vi "HFRR ADV v013 new software.vi"() -> ()   [LabVIEW 2025] (continued)
              tunnel: [w2197] -> w2113 mode=indexing
              tunnel: [w2196] -> w2106 mode=indexing
              tunnel: w2150 -> [_]
              tunnel: [w2185] -> w2111 mode=indexing
              tunnel: [w2190] -> w2108 mode=indexing
              tunnel: [w2186] -> w2098 mode=indexing
              tunnel: [w2181] -> w2073 mode=indexing
              tunnel: [w2177] -> w2054 mode=indexing
              tunnel: [w2172] -> w2014 mode=indexing
              (unwired) 1.0 ("x")
              (unwired) TRUE ("line mode (F)")
              n2047 = Read from Text File "Read File"(file (use dialog)=w2208, error in=w2207) -> (text=w2173:string)  [unwired: 2 in, 3 out]
              n2048 = local write "String 12"(w2173) -> ()
              n2049 = String Subset(string=w2173, offset (0)=85, length (rest)=9 ("length (rest)")) -> (substring=w2175:string)
              n2050 = String Subset(string=w2173, offset (0)=35, length (rest)=9 ("length (rest)")) -> (substring=w2198:string)
              n2051 = String Subset(string=w2173, offset (0)=55, length (rest)=9 ("length (rest)")) -> (substring=w2183:string)
              n2052 = String Subset(string=w2173, offset (0)=25, length (rest)=9 ("length (rest)")) -> (substring=w2179:string)
              n2053 = String Subset(string=w2173, offset (0)=45, length (rest)=9 ("length (rest)")) -> (substring=w2188:string)
              n2054 = String Subset(string=w2173, offset (0)=15, length (rest)=9 ("length (rest)")) -> (substring=w2204:string)
              n2055 = String Subset(string=w2173, offset (0)=0, length (rest)=14 ("length (rest)")) -> (substring=w2201:string)
              n2056 = String Subset(string=w2173, offset (0)=65, length (rest)=9 ("length (rest)")) -> (substring=w2191:string)
              n2057 = Fract/Exp String To Number(string=w2175) -> (number=w2172:dbl)  [unwired: 3 in, 1 out]
              n2058 = Fract/Exp String To Number(string=w2198) -> (number=w2196:dbl)  [unwired: 3 in, 1 out]
              n2059 = Fract/Exp String To Number(string=w2183) -> (number=w2181:dbl)  [unwired: 3 in, 1 out]
              n2060 = Fract/Exp String To Number(string=w2179) -> (number=w2177:dbl)  [unwired: 3 in, 1 out]
              n2061 = Fract/Exp String To Number(string=w2188) -> (number=w2186:dbl)  [unwired: 3 in, 1 out]
              n2062 = Fract/Exp String To Number(string=w2204) -> (number=w2185:dbl)  [unwired: 3 in, 1 out]
              n2063 = Fract/Exp String To Number(string=w2201) -> (number=w2197:dbl)  [unwired: 3 in, 1 out]
              n2064 = Fract/Exp String To Number(string=w2191) -> (number=w2194:dbl)  [unwired: 3 in, 1 out]
              n2065 = Add(x=w2194, y=0.0) -> (x+y=w2190:dbl)
            }
            n2066 = Delete From Array(array=w2056, index=0) -> (array with subset deleted=w2029:dbl[])  [unwired: 1 in, 1 out]
            n2067 = Delete From Array(array=w2119, index=0) -> (array with subset deleted=w2092:dbl[])  [unwired: 1 in, 1 out]
            n2068 = Delete From Array(array=w2099, index=0) -> (array with subset deleted=w2087:dbl[])  [unwired: 1 in, 1 out]
            n2069 = Delete From Array(array=w2117, index=0) -> (array with subset deleted=w2118:dbl[])  [unwired: 1 in, 1 out]
            n2070 = call-poly <vilib>:"Mean.vi"("X"=w2029) -> ("mean"=→"КОФ2 4":dbl)  [unwired: 1 out]
            n2071 = call-poly <vilib>:"Mean.vi"("X"=w2092) -> ("mean"=→"КОФ3":dbl)  [unwired: 1 out]
            n2072 = call-poly <vilib>:"Mean.vi"("X"=w2087) -> ("mean"=→"CP3":dbl)  [unwired: 1 out]
            n2073 = Delete From Array(array=w2081, index=0) -> (array with subset deleted=w2008:dbl[])  [unwired: 1 in, 1 out]
            n2074 = Delete From Array(array=w2020, index=0) -> (array with subset deleted=w2007:dbl[])  [unwired: 1 in, 1 out]
            n2075 = Delete From Array(array=w2060, index=0) -> (array with subset deleted=w2031:dbl[])  [unwired: 1 in, 1 out]
            n2076 = Delete From Array(array=w2138, index=0) -> (array with subset deleted=w2093:dbl[])  [unwired: 1 in, 1 out]
            n2077 = Delete From Array(array=w2104, index=0) -> (array with subset deleted=w2089:dbl[])  [unwired: 1 in, 1 out]
            "array w/ subset deleted" <- w2089
            n2078 = Delete From Array(array=w2135, index=0) -> (array with subset deleted=w2136:dbl[])  [unwired: 1 in, 1 out]
            n2079 = call-poly <vilib>:"Mean.vi"("X"=w2031) -> ("mean"=→"КОФ2 2":dbl)  [unwired: 1 out]
            n2080 = call-poly <vilib>:"Mean.vi"("X"=w2093) -> ("mean"=→"КОФ1":dbl)  [unwired: 1 out]
            n2081 = Bundle "Bundle"(w2008, w2007) -> (w2013:cluster{dbl[], dbl[]})  [unwired: 1 in]
            n2082 = Bundle "Bundle"(w2008, w2136) -> (w2000:cluster{dbl[], dbl[]})  [unwired: 1 in]
            n2083 = Delete From Array(array=w2015, index=0) -> (array with subset deleted=w2003:dbl[])  [unwired: 1 in, 1 out]
            n2084 = Delete From Array(array=w2016, index=0) -> (array with subset deleted=w2005:dbl[])  [unwired: 1 in, 1 out]
            n2085 = Delete From Array(array=w2126, index=0) -> (array with subset deleted=w2127:dbl[])  [unwired: 1 in, 1 out]
            n2086 = Delete From Array(array=w2014, index=0) -> (array with subset deleted=w2001:dbl[])  [unwired: 1 in, 1 out]
            n2087 = Delete From Array(array=w2108, index=0) -> (array with subset deleted=w2109:dbl[])  [unwired: 1 in, 1 out]
            n2088 = Delete From Array(array=w2133, index=0) -> (array with subset deleted=w2039:dbl[])  [unwired: 1 in, 1 out]
            n2089 = Delete From Array(array=w2079, index=0) -> (array with subset deleted=w2035:dbl[])  [unwired: 1 in, 1 out]
            n2090 = Delete From Array(array=w2115, index=0) -> (array with subset deleted=w2037:dbl[])  [unwired: 1 in, 1 out]
            n2091 = Delete From Array(array=w2075, index=0) -> (array with subset deleted=w2033:dbl[])  [unwired: 1 in, 1 out]
            n2092 = Delete From Array(array=w2124, index=0) -> (array with subset deleted=w2038:dbl[])  [unwired: 1 in, 1 out]
            n2093 = Delete From Array(array=w2077, index=0) -> (array with subset deleted=w2034:dbl[])  [unwired: 1 in, 1 out]
            n2094 = Delete From Array(array=w2058, index=0) -> (array with subset deleted=w2030:dbl[])  [unwired: 1 in, 1 out]
            n2095 = Delete From Array(array=w2102, index=0) -> (array with subset deleted=w2088:dbl[])  [unwired: 1 in, 1 out]
            n2096 = Delete From Array(array=w2129, index=0) -> (array with subset deleted=w2090:dbl[])  [unwired: 1 in, 1 out]
            n2097 = Delete From Array(array=w2106, index=0) -> (array with subset deleted=w2036:dbl[])  [unwired: 1 in, 1 out]
            n2098 = Delete From Array(array=w2073, index=0) -> (array with subset deleted=w2032:dbl[])  [unwired: 1 in, 1 out]
            n2099 = Delete From Array(array=w2054, index=0) -> (array with subset deleted=w2028:dbl[])  [unwired: 1 in, 1 out]
            n2100 = Delete From Array(array=w2098, index=0) -> (array with subset deleted=w2086:dbl[])  [unwired: 1 in, 1 out]
            n2101 = Delete From Array(array=w2111, index=0) -> (array with subset deleted=w2091:dbl[])  [unwired: 1 in, 1 out]
            n2102 = Delete From Array(array=w2121, index=0) -> (array with subset deleted=w2004:dbl[])  [unwired: 1 in, 1 out]
            n2103 = Delete From Array(array=w2131, index=0) -> (array with subset deleted=w2006:dbl[])  [unwired: 1 in, 1 out]
            n2104 = Delete From Array(array=w2113, index=0) -> (array with subset deleted=w2002:dbl[])  [unwired: 1 in, 1 out]
            n2105 = Bundle "Bundle"(w2008, w2039) -> (w2026:cluster{dbl[], dbl[]})  [unwired: 1 in]
            n2106 = Bundle "Bundle"(w2008, w2093) -> (w2027:cluster{dbl[], dbl[]})  [unwired: 1 in]
            n2107 = Bundle "Bundle"(w2039, w2035) -> (w2041:cluster{dbl[], dbl[]})  [unwired: 1 in]
            n2108 = Bundle "Bundle"(w2004, w2003) -> (w2011:cluster{dbl[], dbl[]})  [unwired: 1 in]
            n2109 = Bundle "Bundle"(w2037, w2033) -> (w2043:cluster{dbl[], dbl[]})  [unwired: 1 in]
            n2110 = Bundle "Bundle"(w2004, w2037) -> (w2147:cluster{dbl[], dbl[]})  [unwired: 1 in]
            n2111 = Bundle "Bundle"(w2004, w2033) -> (w2071:cluster{dbl[], dbl[]})  [unwired: 1 in]
            n2112 = Bundle "Bundle"(w2004, w2092) -> (w2157:cluster{dbl[], dbl[]})  [unwired: 1 in]
            n2113 = Bundle "Bundle"(w2004, w2087) -> (w2095:cluster{dbl[], dbl[]})  [unwired: 1 in]
            n2114 = Bundle "Bundle"(w2004, w2118) -> (w2142:cluster{dbl[], dbl[]})  [unwired: 1 in]
            n2115 = Bundle "Bundle"(w2038, w2034) -> (w2042:cluster{dbl[], dbl[]})  [unwired: 1 in]
            n2116 = Bundle "Bundle"(w2006, w2005) -> (w2012:cluster{dbl[], dbl[]})  [unwired: 1 in]
            n2117 = Bundle "Bundle"(w2006, w2038) -> (w2149:cluster{dbl[], dbl[]})  [unwired: 1 in]
            n2118 = Bundle "Bundle"(w2006, w2034) -> (w2072:cluster{dbl[], dbl[]})  [unwired: 1 in]
            n2119 = Bundle "Bundle"(w2006, w2088) -> (w2096:cluster{dbl[], dbl[]})  [unwired: 1 in]
            n2120 = Bundle "Bundle"(w2006, w2090) -> (w2158:cluster{dbl[], dbl[]})  [unwired: 1 in]
            n2121 = Bundle "Bundle"(w2006, w2127) -> (w2140:cluster{dbl[], dbl[]})  [unwired: 1 in]
            n2122 = Bundle "Bundle"(w2036, w2032) -> (w2044:cluster{dbl[], dbl[]})  [unwired: 1 in]
            n2123 = Bundle "Bundle"(w2002, w2001) -> (w2010:cluster{dbl[], dbl[]})  [unwired: 1 in]
            n2124 = Bundle "Bundle"(w2002, w2036) -> (w2148:cluster{dbl[], dbl[]})  [unwired: 1 in]
            n2125 = Bundle "Bundle"(w2002, w2032) -> (w2070:cluster{dbl[], dbl[]})  [unwired: 1 in]
            n2126 = Bundle "Bundle"(w2002, w2086) -> (w2094:cluster{dbl[], dbl[]})  [unwired: 1 in]
            n2127 = Bundle "Bundle"(w2002, w2091) -> (w2156:cluster{dbl[], dbl[]})  [unwired: 1 in]
            n2128 = Bundle "Bundle"(w2002, w2109) -> (w2141:cluster{dbl[], dbl[]})  [unwired: 1 in]
            n2129 = call-poly <vilib>:"Mean.vi"("X"=w2089) -> ("mean"=→"CP1":dbl)  [unwired: 1 out]
            n2130 = call-poly <vilib>:"Mean.vi"("X"=w2030) -> ("mean"=→"КОФ2 3":dbl)  [unwired: 1 out]
            n2131 = call-poly <vilib>:"Mean.vi"("X"=w2088) -> ("mean"=→"CP2":dbl)  [unwired: 1 out]
            n2132 = call-poly <vilib>:"Mean.vi"("X"=w2090) -> ("mean"=→"КОФ2":dbl)  [unwired: 1 out]
            n2133 = call-poly <vilib>:"Mean.vi"("X"=w2028) -> ("mean"=→"КОФ2 5":dbl)  [unwired: 1 out]
            n2134 = call-poly <vilib>:"Mean.vi"("X"=w2086) -> ("mean"=→"CP4":dbl)  [unwired: 1 out]
            n2135 = call-poly <vilib>:"Mean.vi"("X"=w2091) -> ("mean"=→"КОФ4":dbl)  [unwired: 1 out]
            n2136 = Bundle "Bundle"(w2008, w2035) -> (w1999:cluster{dbl[], dbl[]})  [unwired: 1 in]
            n2137 = Bundle "Bundle"(w2008, w2089) -> (w2022:cluster{dbl[], dbl[]})  [unwired: 1 in]
            n2138 = Build Array "Build Array"(w1999, w2022) -> (w2025:cluster{dbl[], dbl[]}[])
            "XY Graph 17" <- w2025
            n2139 = Build Array "Build Array"(w2013, w2012, w2011, w2010) -> (→"Frequency ( Hz )":cluster{dbl[], dbl[]}[])
            n2140 = Build Array "Build Array"(w2041, w2042, w2043, w2044) -> (→"Air Temp ( °C ) vs Humidity ( % RH )":cluster{dbl[], dbl[]}[])
            n2141 = Build Array "Build Array"(w2026, w2149, w2147, w2148) -> (→"Air Temperature  ( °C )":cluster{dbl[], dbl[]}[])
            n2142 = Build Array "Build Array"(w1999, w2072, w2071, w2070) -> (→"Humidity ( %RH )":cluster{dbl[], dbl[]}[])
            n2143 = Build Array "Build Array"(w2027, w2158, w2157, w2156) -> (→"Coefficient Of Friction":cluster{dbl[], dbl[]}[])
            n2144 = Build Array "Build Array"(w2022, w2096, w2095, w2094) -> (→"Sample Temperature ( °C )":cluster{dbl[], dbl[]}[])
            n2145 = Build Array "Build Array"(w2000, w2140, w2142, w2141) -> (→"XY Graph 13":cluster{dbl[], dbl[]}[])
            n2146 = Bundle "Bundle"(w2008, w2031) -> (w2053:cluster{dbl[], dbl[]})  [unwired: 1 in]
            n2147 = Bundle "Bundle"(w2004, w2029) -> (w2051:cluster{dbl[], dbl[]})  [unwired: 1 in]
            n2148 = Bundle "Bundle"(w2006, w2030) -> (w2052:cluster{dbl[], dbl[]})  [unwired: 1 in]
            n2149 = Bundle "Bundle"(w2002, w2028) -> (w2050:cluster{dbl[], dbl[]})  [unwired: 1 in]
            n2150 = Build Array "Build Array"(w2053, w2052, w2051, w2050) -> (→"Stroke ( mm )":cluster{dbl[], dbl[]}[])
            n2151 = local write "XY Graph 16"(w2025) -> ()
          }
          frame #2 {
          }
          frame #3 {
            n2152 = local write "Numeric 8"(0 ("Numeric 8")) -> ()
            n2153 = local write "Numeric 11"(0 ("Numeric 11")) -> ()
            n2154 = local write "Numeric 12"(0 ("Numeric 12")) -> ()
            n2155 = local write "Numeric 13"(0 ("Numeric 13")) -> ()
            n2156 = property on="OPEN" class="Bool (strict)"("Visible"=TRUE) -> ()  [unwired: 2 in, 2 out]
            n2157 = local read "String Control 2"() -> (w2325:string)
            n2158 = local read "String Control 4"() -> (w2324:string)
            n2159 = local read "String Control 6"() -> (w2323:string)
            n2160 = local read "String Control 8"() -> (w2322:string)
            n2161 = Match Pattern(string=w2325, regular expression="Samples / cycle :- ") -> (after substring=w2339:string)  [unwired: 1 in, 3 out]
            n2162 = Match Pattern(string=w2325, regular expression="Frequency :- ") -> (after substring=w2358:string)  [unwired: 1 in, 3 out]
            n2163 = Match Pattern(string=w2324, regular expression="Samples / cycle :- ") -> (after substring=w2335:string)  [unwired: 1 in, 3 out]
            n2164 = Match Pattern(string=w2324, regular expression="Frequency :- ") -> (after substring=w2353:string)  [unwired: 1 in, 3 out]
            n2165 = Match Pattern(string=w2323, regular expression="Samples / cycle :- ") -> (after substring=w2331:string)  [unwired: 1 in, 3 out]
            n2166 = Match Pattern(string=w2323, regular expression="Frequency :- ") -> (after substring=w2348:string)  [unwired: 1 in, 3 out]
            n2167 = Match Pattern(string=w2322, regular expression="Samples / cycle :- ") -> (after substring=w2327:string)  [unwired: 1 in, 3 out]
            n2168 = Match Pattern(string=w2322, regular expression="Frequency :- ") -> (after substring=w2343:string)  [unwired: 1 in, 3 out]
            n2169 = String Subset(string=w2339, length (rest)=6 ("length (rest)")) -> (substring=w2341:string)  [unwired: 1 in]
            n2170 = String Subset(string=w2358, length (rest)=9 ("length (rest)")) -> (substring=w2360:string)  [unwired: 1 in]
            n2171 = String Subset(string=w2335, length (rest)=6 ("length (rest)")) -> (substring=w2337:string)  [unwired: 1 in]
            n2172 = String Subset(string=w2353, length (rest)=9 ("length (rest)")) -> (substring=w2355:string)  [unwired: 1 in]
            n2173 = String Subset(string=w2331, length (rest)=6 ("length (rest)")) -> (substring=w2333:string)  [unwired: 1 in]
            n2174 = String Subset(string=w2348, length (rest)=9 ("length (rest)")) -> (substring=w2350:string)  [unwired: 1 in]
            n2175 = String Subset(string=w2327, length (rest)=6 ("length (rest)")) -> (substring=w2329:string)  [unwired: 1 in]
            n2176 = String Subset(string=w2343, length (rest)=9 ("length (rest)")) -> (substring=w2345:string)  [unwired: 1 in]
            n2177 = Fract/Exp String To Number(string=w2341) -> (number=w2321:dbl)  [unwired: 3 in, 1 out]
            n2178 = Fract/Exp String To Number(string=w2360) -> (number=w2361:dbl)  [unwired: 3 in, 1 out]
            n2179 = Fract/Exp String To Number(string=w2337) -> (number=w2320:dbl)  [unwired: 3 in, 1 out]
            n2180 = Fract/Exp String To Number(string=w2355) -> (number=w2356:dbl)  [unwired: 3 in, 1 out]
            n2181 = Fract/Exp String To Number(string=w2333) -> (number=w2319:dbl)  [unwired: 3 in, 1 out]
            n2182 = Fract/Exp String To Number(string=w2350) -> (number=w2351:dbl)  [unwired: 3 in, 1 out]
            n2183 = Fract/Exp String To Number(string=w2329) -> (number=w2318:dbl)  [unwired: 3 in, 1 out]
            n2184 = Fract/Exp String To Number(string=w2345) -> (number=w2346:dbl)  [unwired: 3 in, 1 out]
            n2185 = local write "sample1"(w2321) -> ()
            n2186 = local write "freq1"(w2361) -> ()
            n2187 = local write "sample2"(w2320) -> ()
            n2188 = local write "freq2"(w2356) -> ()
            n2189 = local write "sample3"(w2319) -> ()
            n2190 = local write "freq3"(w2351) -> ()
            n2191 = local write "sample4"(w2318) -> ()
            n2192 = local write "freq 4"(w2346) -> ()
          }
        }
      }
    }
    n2193 = case shown="True" w1810 {
      selector: w1810 -> [_ w1938]
      frame False {
      }
      frame True {
        n2194 = Not(x=w1938) -> (.not. x?=w1934:bool)
        n2195 = local write "service 3"(w1934) -> ()
        n2196 = local write "OPEN 6"(w1934) -> ()
        n2197 = call <vilib>:"System Exec.vi"("wait until completion? (T)"=TRUE, "command line"="C:\\LAB-IQ\\Scar View.exe") -> ("error out"=→"error out 5":errorcluster)  [unwired: 6 in, 3 out]
      }
    }
    n2198 = case shown="\"Acquire\", Default" w1821 {
      frame "Acquire", Default {
        w2834 = 0.2 ("y")
        w2839 = 1.0 ("y")
        w2840 = 0.8 ("y")
        # "Elapsed time\ncof\nstroke\nAir temp\nTemp\nHumidity"
        n2199 = disable-structure shown="Disabled" {
          frame Disabled {
            n2200 = local read "Flag"() -> (w2857:dbl)
            n2201 = local read "RUN"() -> (w2854:bool)
            n2202 = Not(x=w2854) -> (.not. x?=w2853:bool)
            n2203 = Equal?(x=w2857, y=10.0) -> (x = y?=w2855:bool)
            n2204 = And(x=w2855, y=w2853) -> (x .and. y?=w2852:bool)
            n2205 = case shown="True" w2852 {
              frame False {
              }
              frame True {
                w2858 = FALSE ("Heater Button")
                n2206 = local write "Humidity"(w2858) -> ()
                n2207 = local write "Heater Button"(w2858) -> ()
              }
            }
          }
          frame Enabled {
          }
        }
        n2208 = disable-structure shown="Disabled" {
          frame Disabled {
            n2209 = case shown="True" {
              selector: _ -> [_ _]
              frame False {
              }
              frame True {
                w2949 = TRUE ("Heater")
                n2210 = local write "Humidity"(w2949) -> ()
                n2211 = local write "Heater Button"(w2949) -> ()
                n2212 = local read "TEST STANDARD"() -> (w2952:T3)
                n2213 = local read "TEST STANDARD"() -> (w2947:T3)
                n2214 = Equal?(x=w2952, y=enum16{"ASTM D6079", "ISO 12156", "Custom"}."ISO 12156" ("Test Standard")) -> (x = y?=w2950:bool)
                n2215 = Equal?(x=w2947, y=enum16{"ASTM D6079", "ISO 12156", "Custom"}."ASTM D6079" ("Test Standard")) -> (x = y?=w2946:bool)
                n2216 = case shown="True" w2950 {
                  frame False {
                  }
                  frame True {
                    n2217 = local write "Heater"(TRUE ("Heater")) -> ()
                    n2218 = local write "airtempflg"(FALSE ("airtempflg")) -> ()
                  }
                }
                n2219 = case shown="True" w2946 {
                  frame False {
                  }
                  frame True {
                    n2220 = local write "Heater"(FALSE ("Heater")) -> ()
                    n2221 = local write "airtempflg"(TRUE ("airtempflg")) -> ()
                  }
                }
              }
            }
          }
          frame Enabled {
          }
        }
        n2222 = stacked-sequence {
          frame #0 {
            n2223 = case shown="True" "RST FF" {
              frame False {
              }
              frame True {
                w3015 = 0.0 ("X Scale.Range:Maximum")
                n2224 = property on="Frictional Force ( N )" class="WFChart (strict)"("XScale.Maximum"=600.0 ("X Scale.Range:Maximum"), "XScale.Minimum"=w3015, "YScale.Maximum"=10.0 ("Y Scale.Range:Maximum"), "YScale.Minimum"=w3015) -> ()  [unwired: 2 in, 2 out]
              }
            }
          }
          frame #1 {
            n2225 = case shown="True" "RST TEMP" {
              frame False {
              }
              frame True {
                n2226 = property on="Temperature ( Deg C )" class="WFChart (strict)"("XScale.Minimum"=0.0 ("X Scale.Range:Minimum"), "XScale.Maximum"=600.0 ("X Scale.Range:Maximum"), "YScale.Minimum"=0.0 ("Y Scale.Range:Minimum"), "YScale.Maximum"=100.0 ("Y Scale.Range:Maximum")) -> ()  [unwired: 2 in, 2 out]
              }
            }
          }
          frame #2 {
            n2227 = case shown="True" "RSTCOF" {
              frame False {
              }
              frame True {
                n2228 = property on="Coefficient of Friction" class="WFChart (strict)"("XScale.Minimum"=0.0 ("X Scale.Range:Minimum"), "XScale.Maximum"=600.0 ("X Scale.Range:Maximum"), "YScale.Maximum"=1.0 ("X Scale.Range:Minimum"), "YScale.Minimum"=0.0 ("X Scale.Range:Minimum")) -> ()  [unwired: 2 in, 2 out]
              }
            }
          }
          frame #3 {
            n2229 = case shown="True" "RSTCOF 2" {
              frame False {
              }
              frame True {
                (unwired) 100.0 ("Y Scale.Range:Maximum")
                (unwired) 0.0 ("Y Scale.Range:Minimum")
                (unwired) 600.0 ("X Scale.Range:Maximum")
                (unwired) 0.0 ("X Scale.Range:Minimum")
              }
            }
          }
          frame #4 {
            n2230 = case shown="True" "RSTCOF 3" {
              frame False {
              }
              frame True {
                n2231 = property on="Electrical Contact Resistance ( % )" class="WFChart (strict)"("XScale.Minimum"=0.0 ("X Scale.Range:Minimum"), "XScale.Maximum"=600.0 ("X Scale.Range:Maximum"), "YScale.Minimum"=0.0 ("Y Scale.Range:Minimum"), "YScale.Maximum"=100.0 ("Y Scale.Range:Maximum")) -> ()  [unwired: 2 in, 2 out]
              }
            }
          }
        }
        n2232 = disable-structure shown="Disabled" {
          frame Disabled {
            n2233 = case shown="True" {
              selector: _ -> [_ _]
              frame False {
              }
              frame True {
                n2234 = local read "zflag 2"() -> (w2916:dbl)
                n2235 = local read "yflag"() -> (w2918:dbl)
                n2236 = Equal?(x=w2918, y=2.0 ("tflag")) -> (x = y?=w2920:bool)
                n2237 = Equal?(x=w2916, y=3.0 ("tflag")) -> (x = y?=w2919:bool)
                n2238 = And(x=w2920, y=w2919) -> (x .and. y?=w2914:bool)
                n2239 = case shown="True" w2914 {
                  frame False {
                  }
                  frame True {
                    w2945 = 0.0 ("zflag")
                    n2240 = local write "zflag"(w2945) -> ()
                    n2241 = local write "zflag 2"(w2945) -> ()
                    n2242 = Delete(path (use dialog)=path "C:/LAB-IQ-NXT/WO 2449 TT.sig" ("file path (dialog if empty)")) -> (deleted path=w2944:path)  [unwired: 4 in, 2 out]
                    n2243 = Delete(path (use dialog)=path "C:/LAB-IQ-NXT/WO 2449 TRH.sig" ("file path (dialog if empty)")) -> (deleted path=w2939:path)  [unwired: 4 in, 2 out]
                    n2244 = local read "SEN.RUN HRS"() -> (w2931:dbl)
                    n2245 = local read "SENSOR TIME"() -> (w2929:dbl)
                    n2246 = call <vilib>:"compatOverwrite.vi"("overwrite (F)"=TRUE) -> ("overwrite?"=w2921:T29)
                    n2247 = call <vilib>:"compatOverwrite.vi"("overwrite (F)"=TRUE) -> ("overwrite?"=w2925:T29)
                    n2248 = local read "Total No. of Tests"() -> (w2932:dbl)
                    n2249 = Add(x=w2929, y=w2931) -> (x+y=w2930:dbl)
                    "SEN.RUN HRS" <- w2930
                    n2250 = Open/Create/Replace File(file path (use dialog)=w2944, operation (0:open)=w2921) -> (refnum out=w2922:refnum<file>, error out=w2923:errorcluster)  [unwired: 4 in, 1 out]
                    n2251 = Open/Create/Replace File(file path (use dialog)=w2939, operation (0:open)=w2925) -> (refnum out=w2926:refnum<file>, error out=w2927:errorcluster)  [unwired: 4 in, 1 out]
                    n2252 = Deny Access(4:w2923, 6:T27."deny none" ("deny mode (2)"), 7:w2922) -> (3:w2943:refnum<file>)  [unwired: 1 out]
                    n2253 = Deny Access(4:w2927, 6:T27."deny none" ("deny mode (2)"), 7:w2926) -> (3:w2935:refnum<file>)  [unwired: 1 out]
                    n2254 = Number To Decimal String(number=w2932) -> (decimal integer string=w2940:string)  [unwired: 1 in]
                    n2255 = Number To Decimal String(number=w2930) -> (decimal integer string=w2936:string)  [unwired: 1 in]
                    n2256 = Write to Binary File(file (use dialog)=w2943, data=w2940, 5:FALSE ("prepend array or string size? (T)")) -> ()  [unwired: 3 in, 3 out]
                    n2257 = Write to Binary File(file (use dialog)=w2935, data=w2936, 5:FALSE ("prepend array or string size? (T)")) -> ()  [unwired: 3 in, 3 out]
                  }
                }
              }
            }
          }
          frame Enabled {
          }
        }
        n2258 = local read "RUN"() -> (w2843:bool)
        n2259 = local read "run replace"() -> (w2847:bool)
        n2260 = local read "run replace"() -> (w2846:bool)
        n2261 = case shown="True" w2843 {
          frame False {
            n2262 = local write "run replace"(FALSE ("run replace")) -> ()
          }
          frame True {
            "run replace" <- TRUE ("run replace")
          }
        }
        n2263 = local read "RUN"() -> (w2851:bool)
        n2264 = local read "Set Temp"() -> (w2813:dbl)
        n2265 = local read "SetTemp"() -> (w2815:dbl)
        n2266 = case shown="False" w2851 {
          tunnel: [FALSE ("TEST RUNNING") TRUE ("TEST RUNNING")] -> w2850
          frame False {
            w3034 = 0.0 ("Flag")
            n2267 = local write "Elapsed time"(0.0 ("elapsedtime")) -> ()
            n2268 = local write "Time Remaining"(w3034) -> ()
            n2269 = local write "Flag"(w3034) -> ()
            n2270 = local write "Remaining Time"(w3034) -> ()
          }
          frame True {
            n2271 = local write "Flag"(10.0 ("Flag")) -> ()
          }
        }
        n2272 = case shown="False" w2847 {
          frame False {
            n2273 = local read "zflag"() -> (→"zflag 2":dbl)
            n2274 = local write "yflag"(2.0 ("tflag")) -> ()
            n2275 = local write "FLAG 4"(0.0 ("FLAG")) -> ()
          }
          frame True {
            n2276 = local write "yflag"(1.0 ("tflag")) -> ()
            n2277 = local write "zflag"(3.0 ("zflag")) -> ()
          }
        }
        n2278 = local read "acq 2"() -> (w2845:bool)
        n2279 = local read "AIR TEMP"() -> (w2808:dbl)
        n2280 = local read "Amb temp"() -> (w2812:dbl)
        n2281 = case shown="True" "Save & Continue" {
          frame False {
          }
          frame True {
            "acq 2" <- TRUE ("acq 2")
          }
        }
        n2282 = local read "Set Rh"() -> (w2814:dbl)
        n2283 = Add(x=w2815, y=w2840) -> (x+y=w2841:dbl)
        n2284 = Subtract(x=w2815, y=w2840) -> (x-y=w2842:dbl)
        n2285 = Add(x=w2813, y=w2834) -> (x+y=w2835:dbl)
        n2286 = Subtract(x=w2813, y=w2834) -> (x-y=w2836:dbl)
        n2287 = And(x=w2845, y=w2846) -> (x .and. y?=w2844:bool)
        n2288 = Greater Or Equal?(x=w2808, y=15.0) -> (x >= y?=w2809:bool)
        "powstat" <- w2809
        n2289 = local read "Humidity ( %RH )"() -> (w2811:dbl)
        n2290 = case shown="True" "Save & Continue" {
          frame False {
          }
          frame True {
            n2291 = while {
              tunnel: "0123456789abcdefghijklmnopqrstuvwxyzABCDEFGHIJKLMNOPQRSTUVWXYZ" ("string 2") -> [w3005]
              shift-right: [w3003] -> w2998
              shift-left: "" -> [w3002]
              i -> [w3012]
              stop <- w3011 stop-if-true
              n2292 = Random Number (0-1)() -> (number: 0 to 1=w3006:dbl)
              n2293 = Multiply(x=w3006, y=62.0) -> (x*y=w3008:dbl)
              n2294 = Decrement(x="Length") -> (x-1=w3001:i16)
              n2295 = To Word Integer(number=w3008) -> (16bit integer=w3009:i16)
              n2296 = String Subset(string=w3005, offset (0)=w3009, length (rest)=1 ("length (rest)")) -> (substring=w3004:string)
              n2297 = Greater Or Equal?(x=w3012, y=w3001) -> (x >= y?=w3011:bool)
              n2298 = Concatenate Strings(w3004, w3002) -> (w3003:string)
            }
            n2299 = local write "UUID"(w2998) -> ()
          }
        }
        n2300 = In Range and Coerce(upper limit=w2841, x=w2812, lower limit=w2842) -> (In Range?=w2831:bool)  [unwired: 1 out]
        n2301 = Add(x=w2814, y=w2839) -> (x+y=w2838:dbl)
        n2302 = Subtract(x=w2814, y=w2839) -> (x-y=w2837:dbl)
        n2303 = local read "TEMP"() -> (w2810:dbl)
        n2304 = case shown="True" "Save & Continue" {
          frame False {
          }
          frame True {
            n2305 = local read "Operator ID"() -> (w3329:string)
            n2306 = local read "FILE"() -> (w3335:string)
            n2307 = String Length(string=w3335) -> (length=w3333:i32)
            n2308 = String Length(string=w3329) -> (length=w3330:i32)
            n2309 = Greater?(x=w3333, y=0) -> (0:w3332:bool)
            n2310 = Greater?(x=w3330, y=0) -> (0:w3328:bool)
            n2311 = And(x=w3332, y=w3328) -> (x .and. y?=w3327:bool)
            n2312 = case shown="True" w3327 {
              frame False {
                n2313 = stacked-sequence {
                  frame #0 {
                    n2314 = One Button Dialog(message="Please Enter a File Name and Operator ID to save data !", button name ("OK")="Ok") -> ()  [unwired: 1 out]
                  }
                  frame #1 {
                    n2315 = local write "Save & Continue"(FALSE ("OK Button")) -> ()
                  }
                }
                n2316 = local write "Save & Continue"(FALSE ("OK Button")) -> ()
              }
              frame True {
                n2317 = stacked-sequence {
                  frame #0 {
                    n2318 = local read "FILE"() -> (w3341:string)
                    n2319 = call "file check.vi"("file name in"=w3341) -> ("file name out"=w3340:string)  [unwired: 9 in, 1 out]
                    n2320 = call <vilib>:"Application Directory.vi"() -> ("Application Directory"=w3351:path)
                    n2321 = Build Path(base path=w3351, name or relative path="data") -> (appended path=w3350:path)
                    n2322 = call <vilib>:"Trim Whitespace.vi"("string"=w3340) -> ("trimmed string"=w3348:string)  [unwired: 1 in]
                    n2323 = call <vilib>:"Trim Whitespace.vi"("string"=w3340) -> ("trimmed string"=w3349:string)  [unwired: 1 in]
                    n2324 = List Folder(path=w3350) -> (folder names=w3346:string[])  [unwired: 3 in, 3 out]
                    n2325 = Match Pattern(string=w3348, regular expression="_(") -> (before substring=w3345:string)  [unwired: 1 in, 3 out]
                    n2326 = for {
                      tunnel: w3346 -> [w3360] mode=indexing
                      tunnel: w3345 -> [w3358]
                      shift-right: [w3356] -> w3343
                      shift-left: bool[] [] -> [w3357]
                      n2327 = Match Pattern(string=w3360, regular expression="_(") -> (before substring=w3359:string)  [unwired: 1 in, 3 out]
                      n2328 = Equal?(x=w3359, y=w3358) -> (x = y?=w3355:bool)
                      n2329 = case shown="True" w3355 {
                        tunnel: w3355 -> [_ w3363]
                        tunnel: w3357 -> [w3362 w3365]
                        tunnel: [w3362 w3364] -> w3356
                        frame False {
                        }
                        frame True {
                          n2330 = Insert Into Array(array=w3365, new element=w3363) -> (w3364:bool[])  [unwired: 1 in]
                        }
                      }
                    }
                    n2331 = Equal?(x=w3346, y=w3345) -> (x = y?=w3354:bool[])
                    n2332 = Or Array Elements(Boolean array=w3354) -> (logical OR=w3353:bool)
                    n2333 = Array Size(array=w3343) -> (size(s)=w3342:i32)
                    n2334 = case shown="True" w3353 {
                      tunnel: w3349 -> [_ w3373]
                      tunnel: w3342 -> [_ w3366]
                      frame False {
                      }
                      frame True {
                        n2335 = Number To Decimal String(number=w3366) -> (decimal integer string=w3369:string)  [unwired: 1 in]
                        n2336 = Search/Split String(string=w3373, search string/char (-)="_(" ("regular expression")) -> (substring before match=w3371:string)  [unwired: 1 in, 2 out]
                        n2337 = Concatenate Strings(w3371, "_(" ("regular expression"), w3369, ")" ("regular expression")) -> (w3367:string)
                        n2338 = local write "FILE"(w3367) -> ()
                      }
                    }
                  }
                  frame #1 {
                    w3375 = 0.0
                    w3388 = cluster{"y":dbl, dbl, "y":dbl}[] [] ("History Data")
                    w3389 = FALSE ("Heater Button")
                    (unwired) ")!" ("string")
                    (unwired) ")" ("string")
                    w3387 = dbl[] [] ("History Data")
                    w3393 = "\r"
                    # "C:\\WinDucom\\Data\\"
                    # "C:\\LAB-IQ-NXT\\data"
                    n2339 = local write "Humidity ( %RH )"(w3375) -> ()
                    n2340 = local write "Frequency ( Hz )"(w3375) -> ()
                    n2341 = local write "Stroke 3"(w3375) -> ()
                    n2342 = local write "speedop"(0.0 ("PIDclk 2")) -> ()
                    n2343 = local write "Set Temp 2"(65.0 ("Set Temp 2")) -> ()
                    n2344 = local write "AIR TEMP"(w3375) -> ()
                    n2345 = local write "clk"(0.0 ("clk")) -> ()
                    n2346 = local write "Stroke 4"(w3375) -> ()
                    n2347 = local write "COF 2"(w3375) -> ()
                    n2348 = local write "TEMP"(w3375) -> ()
                    n2349 = local write "ecr 3"(w3375) -> ()
                    n2350 = local write "FF 3"(w3375) -> ()
                    n2351 = local write "FF 2"(w3375) -> ()
                    n2352 = property on="Humidity ( %RH )" class="WFChart (strict)"("History Data"=w3387) -> ()  [unwired: 2 in, 2 out]
                    n2353 = property on="Coefficient of Friction" class="WFChart (strict)"("History Data"=w3387) -> ()  [unwired: 2 in, 2 out]
                    n2354 = property on="Coefficient of Friction" class="WFChart (strict)"("History Data"=w3387) -> ()  [unwired: 2 in, 2 out]
                    n2355 = property on="Frictional Force ( N )" class="WFChart (strict)"("History Data"=w3387) -> ()  [unwired: 2 in, 2 out]
                    n2356 = property on="Electrical Contact Resistance ( % )" class="WFChart (strict)"("History Data"=w3387) -> ()  [unwired: 2 in, 2 out]
                    n2357 = property on="Electrical Contact Resistance ( % )" class="WFChart (strict)"("History Data"=w3387) -> ()  [unwired: 2 in, 2 out]
                    n2358 = property on="Temperature ( Deg C )" class="WFChart (strict)"("History Data"=w3387) -> ()  [unwired: 2 in, 2 out]
                    n2359 = property on="Frictional Force ( N )" class="WFChart (strict)"("History Data"=w3387) -> ()  [unwired: 2 in, 2 out]
                    n2360 = property on="Coefficient of Friction" class="WFChart (strict)"("History Data"=w3387) -> ()  [unwired: 2 in, 2 out]
                    n2361 = property on="Frictional Force ( N )" class="WFChart (strict)"("History Data"=w3387) -> ()  [unwired: 2 in, 2 out]
                    n2362 = property on="Electrical Contact Resistance ( % )" class="WFChart (strict)"("History Data"=w3387) -> ()  [unwired: 2 in, 2 out]
                    n2363 = property on="Temperature ( Deg C )" class="WFChart (strict)"("History Data"=w3387) -> ()  [unwired: 2 in, 2 out]
                    n2364 = property on="Humidity ( %RH )" class="WFChart (strict)"("History Data"=w3387) -> ()  [unwired: 2 in, 2 out]
                    n2365 = property on="Stroke ( mm )" class="WFChart (strict)"("History Data"=w3388) -> ()  [unwired: 2 in, 2 out]
                    n2366 = property on="Stroke ( mm )" class="WFChart (strict)"("History Data"=w3388) -> ()  [unwired: 2 in, 2 out]
                    n2367 = local write "Humidity"(w3389) -> ()
                    n2368 = local write "Heater Button"(w3389) -> ()
                    n2369 = local read "FILE"() -> (w3383:string)
                    n2370 = disable-structure shown="Enabled" {
                      disable-tunnel: [w3428 _] -> w3374
                      frame Enabled {
                        n2371 = local read "NORMAL LOAD"() -> (w3428:dbl)
                      }
                      frame Disabled {
                      }
                    }
                    n2372 = call "file check.vi"("file name in"=w3383) -> ("error out"=w3386:errorcluster, "file name out"=w3380:string)  [unwired: 9 in]
                    n2373 = call "FILE PATH CREATION.vi"("error in"=w3386, "FILE NAME :"=w3380) -> ("FILE OUT"=w3379:path)  [unwired: 8 in, 1 out]
                    n2374 = Concatenate Strings(w3380, ".dgf" ("Substring")) -> (w3385:string)
                    n2375 = Concatenate Strings(w3380, ".duf" ("Substring")) -> (w3381:string)
                    n2376 = Multiply(x=w3374, y=1.0) -> (x*y=w3407:dbl)
                    n2377 = Build Path(base path=w3379, name or relative path=w3385) -> (appended path=w3378:path)
                    n2378 = Build Path(base path=w3379, name or relative path=w3381) -> (appended path=w3377:path)
                    n2379 = Number To Fractional String(number=w3407, width (-)=i16 5, precision (6)=i16 2) -> (F-format string=w3415:string)  [unwired: 1 in]
                    n2380 = local read "Fuel Discription :"() -> (w3403:string)
                    n2381 = local read "Batch Ref Num :"() -> (w3391:string)
                    n2382 = Get Date/Time String(date format (0)=enum16{"short", "long", "abbreviated"}."short") -> (date string=w3426:string, time string=w3423:string)  [unwired: 2 in]
                    n2383 = local read "Remarks :"() -> (w3402:string)
                    n2384 = Concatenate Strings("Load :- " ("Substring"), w3415, " grams ," ("Substring")) -> (w3414:string)
                    n2385 = local read "String 41"() -> (w3394:string)
                    n2386 = Concatenate Strings(w3403) -> (w3404:string)
                    n2387 = Concatenate Strings(w3391) -> (w3390:string)
                    n2388 = Concatenate Strings("tested by") -> (w3398:string)
                    n2389 = Concatenate Strings("(" ("Substring"), w3426, ")" ("Substring"), w3423) -> (w3396:string)
                    "concatenated string" <- w3396
                    n2390 = Concatenate Strings(w3402, "," ("string")) -> (w3401:string)
                    n2391 = Concatenate Strings("  TIME;      COF;       STROKE;     AIR TEMP;  TEMP;  HUMIDITY;  ECR; PID-OUT; FREQUENCY" ("Substring"), "\r") -> (w3410:string)
                    n2392 = Concatenate Strings(w3394, w3393, "Fuel Discription :-" ("Substring"), w3404, w3393, w3414, w3393, "Batch Ref Num :-" ("Substring"), w3390, w3393, " Remarks :- " ("Substring"), w3401, w3393, " Date :- " ("Substring"), w3396, w3393, "Tested By :-" ("Substring"), w3398) -> (w3408:string)
                    "REMARKS" <- w3408
                    n2393 = call <vilib>:"Write Characters To File.vi"("append to file? (new file:F)"=FALSE, "character string"=w3410, "file path (dialog if empty)"=w3378) -> ()  [unwired: 2 in, 1 out]
                    n2394 = call <vilib>:"Write Characters To File.vi"("append to file? (new file:F)"=FALSE, "character string"=w3408, "file path (dialog if empty)"=w3377) -> ()  [unwired: 2 in, 1 out]
                  }
                  frame #2 {
                    n2395 = local write "Cycles elapsed"(0 ("Cycles elapsed")) -> ()
                    n2396 = local write "cyclecount"(0 ("cyclecount")) -> ()
                    n2397 = local write "Save & Continue"(FALSE ("OK")) -> ()
                    n2398 = local write "autostrtflg"(TRUE ("autostrtflg")) -> ()
                    n2399 = local write "Save"(FALSE ("Save")) -> ()
                    n2400 = Get Date/Time In Seconds() -> (seconds since 1Jan1904=w3433:timestamp)
                    n2401 = To Double Precision Float(number=w3433) -> (double precision float=w3432:dbl)
                    n2402 = local write "acq timer"(w3432) -> ()
                    n2403 = One Button Dialog(message="Please ensure sample is mounted properly and machine is ready in all aspects for testing !", button name ("OK")="Ok") -> ()  [unwired: 1 out]
                  }
                  frame #3 {
                    n2404 = stacked-sequence {
                      frame #0 {
                        n2405 = local write "Main Dashboard Buttons"(T1."Dashboard" ("Main Dashboard Buttons")) -> ()
                        n2406 = local write "Main Tab"(T2."Acquire" ("Main Tab")) -> ()
                      }
                      frame #1 {
                        n2407 = local write "EVENT LOG"("" ("EVENT LOG")) -> ()
                      }
                      frame #2 {
                        n2408 = Wait (ms)(milliseconds to wait=u32 50) -> ()  [unwired: 1 out]
                      }
                      frame #3 {
                        n2409 = disable-structure shown="Disabled" {
                          frame Disabled {
                            n2410 = local read "EVENT LOG"() -> (w3445:string)
                            n2411 = call "Event Log.vi"("Content"="Test Details", "EVENT LOG"=w3445) -> ("EVENT LOG"=w3444:string)  [unwired: 8 in, 1 out]
                            n2412 = local write "EVENT LOG"(w3444) -> ()
                          }
                          frame Enabled {
                          }
                        }
                      }
                      frame #4 {
                        n2413 = Wait (ms)(milliseconds to wait=u32 50) -> ()  [unwired: 1 out]
                      }
                      frame #5 {
                        n2414 = local read "FILE"() -> (w3447:string)
                        n2415 = Concatenate Strings("File Name :" ("Content"), w3447) -> (w3448:string)
                        n2416 = local read "EVENT LOG"() -> (w3451:string)
                        n2417 = call "Event Log.vi"("Content"=w3448, "EVENT LOG"=w3451) -> ("EVENT LOG"=w3450:string)  [unwired: 8 in, 1 out]
                        n2418 = local write "EVENT LOG"(w3450) -> ()
                      }
                      frame #6 {
                        n2419 = Wait (ms)(milliseconds to wait=u32 50) -> ()  [unwired: 1 out]
                      }
                      frame #7 {
                        n2420 = local read "Batch Ref Num :"() -> (w3453:string)
                        n2421 = Concatenate Strings("Batch Ref No :" ("Content"), w3453) -> (w3454:string)
                        n2422 = local read "EVENT LOG"() -> (w3457:string)
                        n2423 = call "Event Log.vi"("Content"=w3454, "EVENT LOG"=w3457) -> ("EVENT LOG"=w3456:string)  [unwired: 8 in, 1 out]
                        n2424 = local write "EVENT LOG"(w3456) -> ()
                      }
                      frame #8 {
                        n2425 = Wait (ms)(milliseconds to wait=u32 50) -> ()  [unwired: 1 out]
                      }
                      frame #9 {
                        n2426 = local read "tested by"() -> (w3459:string)
                        n2427 = Concatenate Strings("Tested By :" ("Content"), w3459) -> (w3460:string)
                        n2428 = local read "EVENT LOG"() -> (w3463:string)
                        n2429 = call "Event Log.vi"("Content"=w3460, "EVENT LOG"=w3463) -> ("EVENT LOG"=w3462:string)  [unwired: 8 in, 1 out]
                        n2430 = local write "EVENT LOG"(w3462) -> ()
                      }
                      frame #10 {
                        n2431 = Wait (ms)(milliseconds to wait=u32 50) -> ()  [unwired: 1 out]
                      }
                      frame #11 {
                        n2432 = local read "TEST STANDARD"() -> (w3466:T3)
                        n2433 = case shown="\"ASTM D6079\", Default" w3466 {
                          tunnel: ["ASTM D6079" "ISO 12156" "CEC F-096-A-06" "Custom"] -> w3465
                          frame "ASTM D6079", Default {
                          }
                          frame "ISO 12156" {
                          }
                          frame "CEC F-096-A-06" {
                          }
                          frame "Custom" {
                          }
                        }
                        n2434 = Concatenate Strings("Test Standard :" ("Content"), w3465) -> (w3467:string)
                        n2435 = local read "EVENT LOG"() -> (w3470:string)
                        n2436 = call "Event Log.vi"("Content"=w3467, "EVENT LOG"=w3470) -> ("EVENT LOG"=w3469:string)  [unwired: 8 in, 1 out]
                        n2437 = local write "EVENT LOG"(w3469) -> ()
                      }
                      frame #12 {
                        n2438 = Wait (ms)(milliseconds to wait=u32 50) -> ()  [unwired: 1 out]
                      }
                      frame #13 {
                        n2439 = local read "Fuel Discription :"() -> (w3476:string)
                        n2440 = Concatenate Strings("Fuel Description :" ("Content"), w3476) -> (w3477:string)
                        n2441 = local read "EVENT LOG"() -> (w3480:string)
                        n2442 = call "Event Log.vi"("Content"=w3477, "EVENT LOG"=w3480) -> ("EVENT LOG"=w3479:string)  [unwired: 8 in, 1 out]
                        n2443 = local write "EVENT LOG"(w3479) -> ()
                      }
                      frame #14 {
                        n2444 = Wait (ms)(milliseconds to wait=u32 50) -> ()  [unwired: 1 out]
                      }
                      frame #15 {
                        n2445 = local read "Remarks :"() -> (w3482:string)
                        n2446 = Concatenate Strings("Remarks :" ("Content"), w3482) -> (w3483:string)
                        n2447 = local read "EVENT LOG"() -> (w3486:string)
                        n2448 = call "Event Log.vi"("Content"=w3483, "EVENT LOG"=w3486) -> ("EVENT LOG"=w3485:string)  [unwired: 8 in, 1 out]
                        n2449 = local write "EVENT LOG"(w3485) -> ()
                      }
                      frame #16 {
                        n2450 = Wait (ms)(milliseconds to wait=u32 50) -> ()  [unwired: 1 out]
                      }
                      frame #17 {
                        n2451 = local read "Operator ID"() -> (w3488:string)
                        n2452 = Concatenate Strings("Operator ID :" ("Content"), w3488) -> (w3490:string)
                        n2453 = local read "EVENT LOG"() -> (w3492:string)
                        n2454 = call "Event Log.vi"("Content"=w3490, "EVENT LOG"=w3492) -> ("EVENT LOG"=w3491:string)  [unwired: 8 in, 1 out]
                        n2455 = local write "EVENT LOG"(w3491) -> ()
                      }
                      frame #18 {
                        n2456 = Wait (ms)(milliseconds to wait=u32 50) -> ()  [unwired: 1 out]
                      }
                      frame #19 {
                        n2457 = disable-structure shown="Disabled" {
                          frame Disabled {
                            n2458 = local read "EVENT LOG"() -> (w3496:string)
                            n2459 = call "Event Log.vi"("Content"="Test Parameter", "EVENT LOG"=w3496) -> ("EVENT LOG"=w3495:string)  [unwired: 8 in, 1 out]
                            n2460 = local write "EVENT LOG"(w3495) -> ()
                          }
                          frame Enabled {
                          }
                        }
                      }
                      frame #20 {
                        n2461 = Wait (ms)(milliseconds to wait=u32 50) -> ()  [unwired: 1 out]
                      }
                      frame #21 {
                        n2462 = local read "Set Hz"() -> (w3500:dbl)
                        n2463 = Number To Fractional String(number=w3500, precision (6)=i16 2) -> (F-format string=w3499:string)  [unwired: 2 in]
                        n2464 = Concatenate Strings("Set Frequency [Hz] :" ("Content"), w3499) -> (w3502:string)
                        n2465 = local read "EVENT LOG"() -> (w3504:string)
                        n2466 = call "Event Log.vi"("Content"=w3502, "EVENT LOG"=w3504) -> ("EVENT LOG"=w3503:string)  [unwired: 8 in, 1 out]
                        n2467 = local write "EVENT LOG"(w3503) -> ()
                      }
                      frame #22 {
                        n2468 = Wait (ms)(milliseconds to wait=u32 50) -> ()  [unwired: 1 out]
                      }
                      frame #23 {
                        n2469 = local read "NORMAL LOAD"() -> (w3507:dbl)
                        n2470 = Number To Fractional String(number=w3507, precision (6)=i16 2) -> (F-format string=w3508:string)  [unwired: 2 in]
                        n2471 = Concatenate Strings("Applied Load [grams] :" ("Content"), w3508) -> (w3510:string)
                        n2472 = local read "EVENT LOG"() -> (w3512:string)
                        n2473 = call "Event Log.vi"("Content"=w3510, "EVENT LOG"=w3512) -> ("EVENT LOG"=w3511:string)  [unwired: 8 in, 1 out]
                        n2474 = local write "EVENT LOG"(w3511) -> ()
                      }
                      frame #24 {
                        n2475 = Wait (ms)(milliseconds to wait=u32 50) -> ()  [unwired: 1 out]
                      }
                      frame #25 {
                        n2476 = local read "Set Strk"() -> (w3515:dbl)
                        n2477 = Number To Fractional String(number=w3515, precision (6)=i16 2) -> (F-format string=w3516:string)  [unwired: 2 in]
                        n2478 = Concatenate Strings("Set Stroke [mm] :" ("Content"), w3516) -> (w3518:string)
                        n2479 = local read "EVENT LOG"() -> (w3520:string)
                        n2480 = call "Event Log.vi"("Content"=w3518, "EVENT LOG"=w3520) -> ("EVENT LOG"=w3519:string)  [unwired: 8 in, 1 out]
                        n2481 = local write "EVENT LOG"(w3519) -> ()
                      }
                      frame #26 {
                        n2482 = Wait (ms)(milliseconds to wait=u32 50) -> ()  [unwired: 1 out]
                      }
                      frame #27 {
                        n2483 = local read "Set Temp"() -> (w3523:dbl)
                        n2484 = Number To Fractional String(number=w3523, precision (6)=i16 2) -> (F-format string=w3524:string)  [unwired: 2 in]
                        n2485 = Concatenate Strings("Set Temperature [deg C] :" ("Content"), w3524) -> (w3526:string)
                        n2486 = local read "EVENT LOG"() -> (w3528:string)
                        n2487 = call "Event Log.vi"("Content"=w3526, "EVENT LOG"=w3528) -> ("EVENT LOG"=w3527:string)  [unwired: 8 in, 1 out]
                        n2488 = local write "EVENT LOG"(w3527) -> ()
                      }
                      frame #28 {
                        n2489 = Wait (ms)(milliseconds to wait=u32 50) -> ()  [unwired: 1 out]
                      }
                      frame #29 {
                        n2490 = local read "Set Rh"() -> (w3531:dbl)
                        n2491 = Number To Fractional String(number=w3531, precision (6)=i16 2) -> (F-format string=w3532:string)  [unwired: 2 in]
                        n2492 = Concatenate Strings("Set Humidity [%RH] :" ("Content"), w3532) -> (w3534:string)
                        n2493 = local read "EVENT LOG"() -> (w3536:string)
                        n2494 = call "Event Log.vi"("Content"=w3534, "EVENT LOG"=w3536) -> ("EVENT LOG"=w3535:string)  [unwired: 8 in, 1 out]
                        n2495 = local write "EVENT LOG"(w3535) -> ()
                      }
                      frame #30 {
                        n2496 = Wait (ms)(milliseconds to wait=u32 50) -> ()  [unwired: 1 out]
                      }
                      frame #31 {
                        n2497 = local read "test time"() -> (w3539:dbl)
                        n2498 = Number To Fractional String(number=w3539, precision (6)=i16 1) -> (F-format string=w3540:string)  [unwired: 2 in]
                        n2499 = Concatenate Strings("Test Duration [mins] :" ("Content"), w3540) -> (w3542:string)
                        n2500 = local read "EVENT LOG"() -> (w3544:string)
                        n2501 = call "Event Log.vi"("Content"=w3542, "EVENT LOG"=w3544) -> ("EVENT LOG"=w3543:string)  [unwired: 8 in, 1 out]
                        n2502 = local write "EVENT LOG"(w3543) -> ()
                      }
                      frame #32 {
                        w3545 = dbl[] [] ("History Data")
                        w3546 = cluster{"y":dbl, dbl, "y":dbl}[] [] ("History Data")
                        w3547 = FALSE ("Visible")
                        n2503 = property on="Stroke ( mm )" class="WFChart (strict)"("History Data"=w3546) -> ()  [unwired: 2 in, 2 out]
                        n2504 = property on="Humidity ( %RH )" class="WFChart (strict)"("History Data"=w3545) -> ()  [unwired: 2 in, 2 out]
                        n2505 = property on="Temperature ( Deg C )" class="WFChart (strict)"("History Data"=w3545) -> ()  [unwired: 2 in, 2 out]
                        n2506 = property on="Electrical Contact Resistance ( % )" class="WFChart (strict)"("History Data"=w3545) -> ()  [unwired: 2 in, 2 out]
                        n2507 = property on="Coefficient of Friction" class="WFChart (strict)"("History Data"=w3545) -> ()  [unwired: 2 in, 2 out]
                        n2508 = property on="Frictional Force ( N )" class="WFChart (strict)"("History Data"=w3545) -> ()  [unwired: 2 in, 2 out]
                        n2509 = property on="Coefficient of Friction" class="WFChart (strict)"("History Data"=w3545) -> ()  [unwired: 2 in, 2 out]
                        n2510 = property on="Frictional Force ( N )" class="WFChart (strict)"("History Data"=w3545) -> ()  [unwired: 2 in, 2 out]
                        n2511 = property on="Electrical Contact Resistance ( % )" class="WFChart (strict)"("History Data"=w3545) -> ()  [unwired: 2 in, 2 out]
                        n2512 = property on="Humidity ( %RH )" class="WFChart (strict)"("History Data"=w3545) -> ()  [unwired: 2 in, 2 out]
                        n2513 = property on="Stroke ( mm )" class="WFChart (strict)"("History Data"=w3546) -> ()  [unwired: 2 in, 2 out]
                        n2514 = property on="Temperature ( Deg C )" class="WFChart (strict)"("History Data"=w3545) -> ()  [unwired: 2 in, 2 out]
                        n2515 = property on="Service Password Log" class="Str"("Visible"=w3547) -> ()  [unwired: 2 in, 2 out]
                        n2516 = property on="Password 3" class="Clust (strict)"("Visible"=w3547) -> ()  [unwired: 2 in, 2 out]
                      }
                    }
                    "TEST FILE NAM,E SAVED" <- TRUE ("TEST FILE NAM,E SAVED")
                  }
                }
              }
            }
          }
        }
        n2517 = case shown="True" w2844 {
          frame False {
            n2518 = local write "tfalg"(0.0 ("tfalg")) -> ()
          }
          frame True {
            n2519 = local read "tfalg"() -> (w2989:dbl)
            n2520 = Equal?(x=w2989, y=0.0) -> (x = y?=w2990:bool)
            n2521 = case shown="True" w2990 {
              frame False {
              }
              frame True {
                n2522 = local read "Total No. of Tests"() -> (w2993:dbl)
                n2523 = local write "tfalg"(1.0 ("tfalg")) -> ()
                n2524 = local write "acq 2"(FALSE ("acq 2")) -> ()
                n2525 = Wait (ms)(milliseconds to wait=u32 200) -> ()  [unwired: 1 out]
                n2526 = Increment(x=w2993) -> (x+1=w2992:dbl)
                n2527 = local write "Total No. of Tests"(w2992) -> ()
              }
            }
          }
        }
        n2528 = local write "Test \nStatus"(w2850) -> ()
        n2529 = local write "Save"(w2850) -> ()
        n2530 = local read "Main Tab"() -> (w2807:T2)
        n2531 = case shown="True" w2831 {
          tunnel: [FALSE ("RUN") TRUE ("RUN")] -> w2830
          tunnel: [_ 1] -> w2823
          frame False {
          }
          frame True {
          }
        }
        n2532 = In Range and Coerce(upper limit=w2838, x=w2811, lower limit=w2837) -> (In Range?=w2829:bool)  [unwired: 1 out]
        n2533 = In Range and Coerce(upper limit=w2835, x=w2810, lower limit=w2836) -> (In Range?=w2827:bool)  [unwired: 1 out]
        n2534 = case shown="True" w2843 {
          frame False {
            n2535 = local read "Rt 3"() -> (w2971:bool)
            n2536 = case shown="True" w2971 {
              frame False {
              }
              frame True {
                n2537 = local write "Rt 3"(FALSE ("Rt 3")) -> ()
                n2538 = local write "Json End Flg"(TRUE ("Upld AR 2")) -> ()
              }
            }
            "Rt" <- TRUE ("Rt")
            "Rt 2" <- FALSE ("Rt")
          }
          frame True {
            n2539 = local read "Rt"() -> (w2978:bool)
            n2540 = local write "Rt 2"(TRUE ("Rt 2")) -> ()
            n2541 = case shown="True" w2978 {
              frame False {
              }
              frame True {
                w2979 = TRUE ("Upld AR 2")
                n2542 = local write "Rt"(FALSE ("Rt")) -> ()
                n2543 = local write "Upld AR"(w2979) -> ()
                n2544 = local write "Json St Flg"(w2979) -> ()
              }
            }
            "Rt 3" <- TRUE ("Rt 3")
          }
        }
        n2545 = case shown="True" w2829 {
          tunnel: [FALSE ("RUN") TRUE ("RUN")] -> w2828
          tunnel: [_ 2] -> w2822
          frame False {
          }
          frame True {
          }
        }
        n2546 = case shown="True" w2827 {
          tunnel: [FALSE ("RUN") TRUE ("RUN")] -> w2826
          tunnel: [_ 3] -> w2821
          frame False {
          }
          frame True {
          }
        }
        n2547 = case shown="\"Acquire\"" w2807 {
          tunnel: w2809 -> [_ w3040]
          frame Default {
            w3039 = 0.0 ("output")
            n2548 = local write "PID-out"(w3039) -> ()
            n2549 = local write "Frequency ( Hz )"(w3039) -> ()
          }
          frame "Acquire" {
            n2550 = stacked-sequence {
              frame #0 {
                n2551 = local read "Auto Start Test"() -> (w3042:bool)
                n2552 = case shown="True" w3042 {
                  tunnel: "RUN" -> [w3063 w3066]
                  tunnel: [w3063 w3065] -> w3043
                  frame False {
                  }
                  frame True {
                    n2553 = local read "Auto Start Temp"() -> (w3064:bool)
                    n2554 = Or(x=w3066, y=w3064) -> (x .or. y?=w3065:bool)
                  }
                }
                n2555 = local read "clk"() -> (w3062:dbl)
                n2556 = local read "Save"() -> (w3058:bool)
                n2557 = Equal?(x=w3062, y=0.0) -> (x = y?=w3059:bool)
                n2558 = And(x=w3059, y=w3058) -> (x .and. y?=w3060:bool)
                n2559 = Not(x="Engage") -> (.not. x?=w3049:bool)
                n2560 = case shown="False" w3043 {
                  tunnel: [0.0 w3089] -> w3045
                  frame False {
                    (unwired) TRUE ("Visible")
                    n2561 = local read "Auto Start Test"() -> (w3070:bool)
                    n2562 = local write "Start Time"(TRUE ("Start Time")) -> ()
                    n2563 = property on="Stroke 2" class="DigNum (strict)"("Visible"=FALSE) -> ()  [unwired: 2 in, 2 out]
                    n2564 = case shown="False" w3070 {
                      frame False {
                        n2565 = property on="Heater Button" class="Bool (strict)"("DisabledEnum"=T17."Enabled" ("Disabled")) -> ()  [unwired: 2 in, 2 out]
                        n2566 = property on="Humidity" class="Bool (strict)"("DisabledEnum"=T17."Enabled" ("Disabled")) -> ()  [unwired: 2 in, 2 out]
                      }
                      frame True {
                      }
                    }
                    n2567 = case shown="False" "TestCompFlg" {
                      frame False {
                        n2568 = local read "StartFlg"() -> (w3078:bool)
                        n2569 = case shown="True" w3078 {
                          frame False {
                          }
                          frame True {
                            n2570 = stacked-sequence {
                              frame #0 {
                                n2571 = local read "EVENT LOG"() -> (w3082:string)
                                n2572 = call "Event Log.vi"("Content"="Test was interrupted", "EVENT LOG"=w3082) -> ("EVENT LOG"=w3083:string)  [unwired: 8 in, 1 out]
                                n2573 = local write "EVENT LOG"(w3083) -> ()
                                n2574 = property on="RUN" class="Bool (strict)"("Visible"=TRUE) -> ()  [unwired: 2 in, 2 out]
                                n2575 = property on="Auto Start Test" class="Bool (strict)"("Visible"=TRUE) -> ()  [unwired: 2 in, 2 out]
                              }
                              frame #1 {
                                w3085 = FALSE ("StartFlg")
                                n2576 = property on="Heater Button" class="Bool (strict)"("Val(Sgnl)"=FALSE ("Value (Signaling)")) -> ()  [unwired: 2 in, 2 out]
                                n2577 = local write "Heater Button"(w3085) -> ()
                                n2578 = local write "StartFlg"(w3085) -> ()
                                n2579 = local write "Humidity"(w3085) -> ()
                              }
                              frame #2 {
                                n2580 = local write "Command"("VC;0" ("Command")) -> ()
                              }
                              frame #3 {
                                n2581 = Wait (ms)(milliseconds to wait=u32 1500) -> ()  [unwired: 1 out]
                              }
